vi "Extended User Data.vi"(7 "Action":u16(ring) items=["Read Data", "Write Data", "Clear Data", "Clear ALL Data"], 8 "error in (no error)":errorcluster, 10 "User Data In":T1, 11 "VISA resource name":refnum<visa-resource-name>) -> (0 "error out":errorcluster, 2 "User Data Out":T1, 3 "VISA resource name out":refnum<visa-resource-name>)   [LabVIEW 2014, in "Agilent PSG MXG Series.lvlib"]
doc: "Writes, reads, and clears data of the type User Data In to the connected VISA session."
uses:
  Agilent PSG MXG Series.lvlib
  Extended User Data.ctl
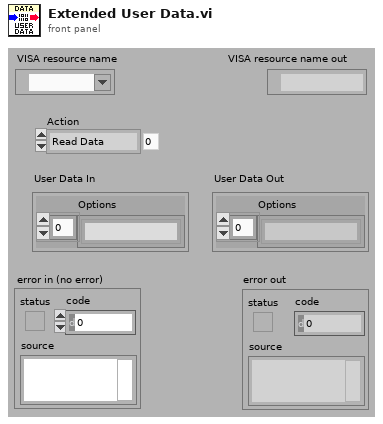
[diagram p1: front panel]
types:
  T1 = typedef "Agilent PSG MXG Series.lvlib/Extended User Data.ctl" = cluster{"Options":string[]}
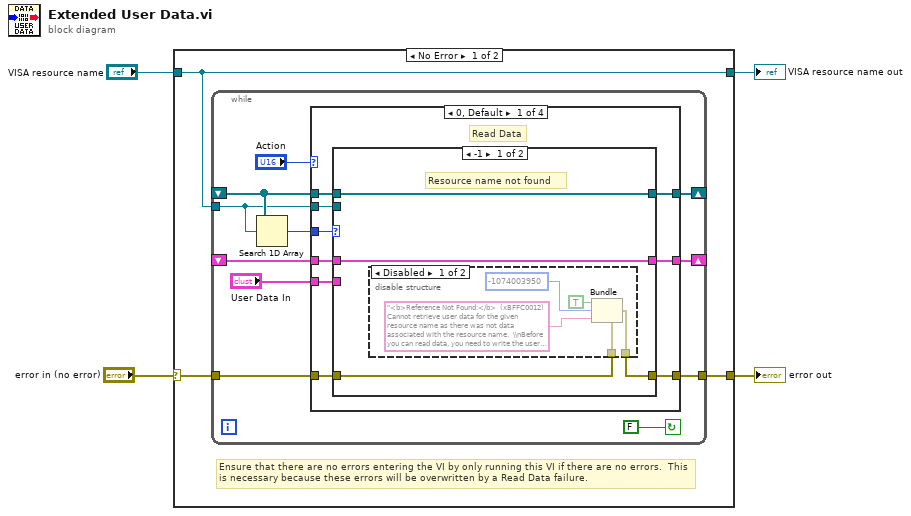
[diagram p0: block diagram]
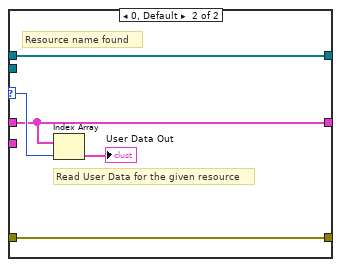
[diagram p3: hidden frame]
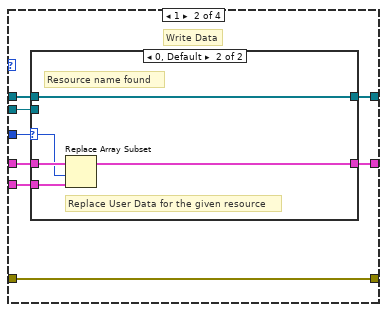
[diagram p4: hidden frame]
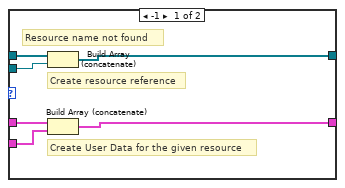
[diagram p5: hidden frame]
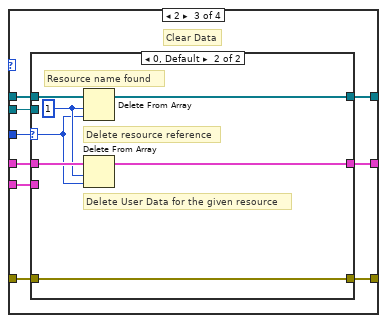
[diagram p6: hidden frame]
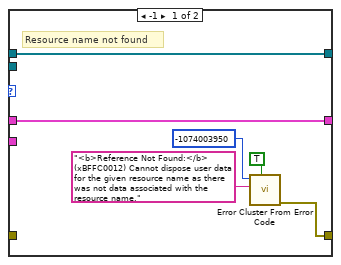
[diagram p7: hidden frame]
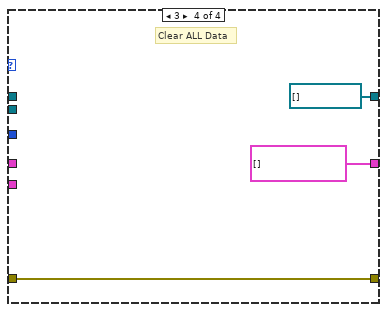
[diagram p8: hidden frame]
diagram:
  n1 = case shown="No Error" "error in (no error)" {
    selector: "error in (no error)" -> [w6 w88]
    tunnel: "VISA resource name" -> [w5 w87]
    tunnel: [w7 w88] -> w3
    tunnel: [w5 w87] -> w1
    frame No Error {
      # "Ensure that there are no errors entering the VI by only running this VI if there are no errors.  This is necessary because these errors will be overwritten by a Read Data failure."
      n2 = while {
        shift-right: [w14] -> _
        shift-left: _ -> [w15]
        shift-right: [w17] -> _
        shift-left: _ -> [w18]
        tunnel: w5 -> [w13]
        tunnel: w6 -> [w10]
        tunnel: [w9] -> w7
        stop <- FALSE continue-if-true
        n3 = Search 1D Array(1D array=w15, element=w13) -> (index of element=w16:i32)  [unwired: 1 out]
        n4 = case shown="0, Default" "Action" {
          tunnel: "User Data In" -> [w27 w50 w70 _]
          tunnel: w18 -> [w26 w49 w69 _]
          tunnel: [w25 w48 w68 T1[] []] -> w17
          tunnel: w16 -> [w24 w47 w67 _]
          tunnel: w15 -> [w23 w46 w66 _]
          tunnel: [w22 w45 w65 refnum<visa-resource-name>[] []] -> w14
          tunnel: w13 -> [w21 w44 w64 _]
          tunnel: w10 -> [w19 w43 w62 w84]
          tunnel: [w20 w43 w63 w84] -> w9
          frame 0, Default {
            # "Read Data"
            n5 = case shown="-1" w24 {
              selector: w24 -> [_ w42]
              tunnel: w27 -> [_ _]
              tunnel: [w30 w39] -> w25
              tunnel: w26 -> [w30 w39]
              tunnel: w23 -> [w31 w41]
              tunnel: [w31 w41] -> w22
              tunnel: w21 -> [_ _]
              tunnel: [w28 w38] -> w20
              tunnel: w19 -> [w29 w38]
              frame -1 {
                # "Resource name not found"
                n6 = disable-structure shown="Disabled" {
                  disable-tunnel: w29 -> [w36 w37]
                  disable-tunnel: [w32 w37] -> w28
                  frame Disabled {
                    n7 = Bundle(cluster=w36, "status"=TRUE ("show call chain? (False)"), "code"=-1074003950 ("Code"), "source"="<b>Reference Not Found:</b>  (xBFFC0012) Cannot retrieve user data for the given resource name as there was not data associated with the resource name.  \\nBefore you can read data, you need to write the user data using the Write Data action of this User Data VI. ") -> (w32:errorcluster)
                  }
                  frame Enabled {
                  }
                }
              }
              frame 0, Default {
                # "Read User Data for the given resource"
                # "Resource name found"
                n8 = Index Array(array=w39, index=w42) -> (element=→"User Data Out":T1)
              }
            }
          }
          frame 1 {
            # "Write Data"
            n9 = case shown="0, Default" w47 {
              selector: w47 -> [_ w58]
              tunnel: w50 -> [w54 w59]
              tunnel: [w53 w61] -> w48
              tunnel: w49 -> [w55 w60]
              tunnel: w46 -> [w56 w57]
              tunnel: [w51 w57] -> w45
              tunnel: w44 -> [w52 _]
              frame -1 {
                # "Create resource reference"
                # "Create User Data for the given resource"
                # "Resource name not found"
                n10 = Build Array (concatenate)(w56, w52) -> (w51:refnum<visa-resource-name>[])
                n11 = Build Array (concatenate)(w55, w54) -> (w53:T1[])
              }
              frame 0, Default {
                # "Replace User Data for the given resource"
                # "Resource name found"
                n12 = Replace Array Subset(array=w60, new element=w59, index=w58) -> (w61:T1[])
              }
            }
          }
          frame 2 {
            # "Clear Data"
            n13 = case shown="0, Default" w67 {
              selector: w67 -> [_ w77]
              tunnel: w70 -> [_ _]
              tunnel: [w75 w83] -> w68
              tunnel: w69 -> [w75 w82]
              tunnel: w66 -> [w76 w80]
              tunnel: [w76 w79] -> w65
              tunnel: w64 -> [_ _]
              tunnel: [w74 w81] -> w63
              tunnel: w62 -> [_ w81]
              frame -1 {
                # "Resource name not found"
                n14 = call "Error Cluster From Error Code.vi"("show call chain? (False)"=TRUE, "error message (\"\")"="<b>Reference Not Found:</b>  (xBFFC0012) Cannot dispose user data for the given resource name as there was not data associated with the resource name.", "error code (0)"=-1074003950 ("Code")) -> ("error out"=w74:errorcluster)  [unwired: 1 in, 5 out]
              }
              frame 0, Default {
                w78 = 1 ("length")
                # "Delete resource reference"
                # "Delete User Data for the given resource"
                # "Resource name found"
                n15 = Delete From Array(array=w80, length=w78, index=w77) -> (array with subset deleted=w79:refnum<visa-resource-name>[])  [unwired: 1 out]
                n16 = Delete From Array(array=w82, length=w78, index=w77) -> (array with subset deleted=w83:T1[])  [unwired: 1 out]
              }
            }
          }
          frame 3 {
            # "Clear ALL Data"
          }
        }
      }
    }
    frame Error {
    }
  }
  "error out" <- w3
  "VISA resource name out" <- w1
